vi "String and values individual array to cluster array.vi"(1 "Value Array In":i32[](array[numeric]), 2 "String Array In":string[](array[string])) -> (0 "Strings and Values Out":T1)   [LabVIEW 2020, in "Basic Fields.lvlib"]
uses:
  <vilib>/Utility/miscctls.llb/LVStringsAndValuesArrayTypeDef.ctl
  Column Libraries/Basic Fields.lvlib
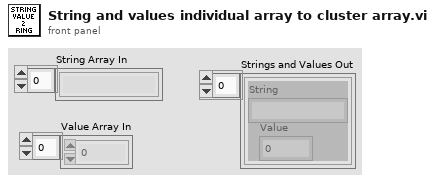
[diagram p1: front panel]
types:
  T1 = typedef "LVStringsAndValuesArrayTypeDef.ctl" = cluster{"String":string, "Value":ext}[]
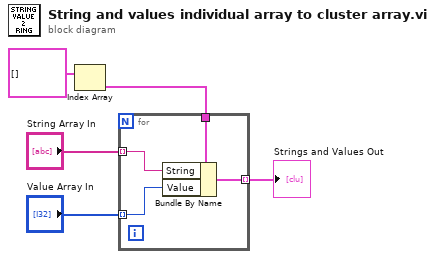
[diagram p0: block diagram]
diagram:
  n1 = Index Array(array=T1 [] ("Strings and Values Out")) -> (element=w4:cluster{"String":string, "Value":ext})  [unwired: 1 in]
  n2 = for {
    tunnel: w4 -> [w9]
    tunnel: "Value Array In" -> [w8] mode=indexing
    tunnel: "String Array In" -> [w7] mode=indexing
    tunnel: [w6] -> w1 mode=indexing
    n3 = Bundle By Name(cluster=w9, "String"=w7, "Value"=w8) -> (w6:cluster{"String":string, "Value":ext})
  }
  "Strings and Values Out" <- w1
